vi "enquece Keypad(SubVI).vi"(6 "priority enquece":bool, 8 "error in (no error)":errorcluster, 9 "keypad cmd":variant, 10 "cmd":string, 11 "Queue in":refnum<queue>) -> (0 "error out":errorcluster, 3 "dup quece":refnum<queue>)   [LabVIEW 2018]
uses:
  project/type defs/test keypad luster.ctl
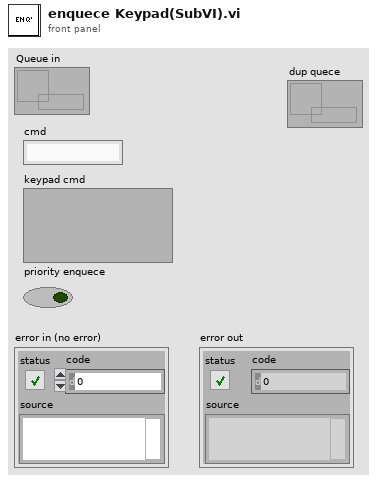
[diagram p1: front panel]
types:
  T1 = typedef "test keypad luster.ctl" = cluster{"cmd":string, "keypad cmd":variant}
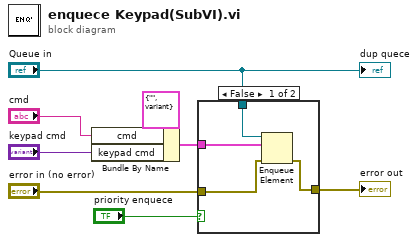
[diagram p0: block diagram]
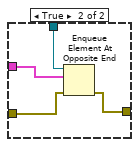
[diagram p2: hidden frame]
diagram:
  n1 = Bundle By Name(cluster=T1 {"cmd"="", "keypad cmd"=variant(refnum<visa-resource-name> "")}, "cmd"="cmd", "keypad cmd"="keypad cmd") -> (w4:T1)
  n2 = case shown="False" "priority enquece" {
    tunnel: [w12 w14] -> w7
    tunnel: "error in (no error)" -> [w11 w15]
    tunnel: "Queue in" -> [w10 w16]
    tunnel: w4 -> [w9 w13]
    frame False {
      n3 = Enqueue Element(queue=w10, element=w9, error in (no error)=w11) -> (error out=w12:errorcluster)  [unwired: 1 in, 2 out]
    }
    frame True {
      n4 = Enqueue Element At Opposite End(queue=w16, element=w13, error in (no error)=w15) -> (error out=w14:errorcluster)  [unwired: 1 in, 2 out]
    }
  }
  "error out" <- w7
  "dup quece" <- "Queue in"
